vi "thermometer.vi"(1 "upper bound":dbl, 2 "lower bound":dbl) -> (0 "Deg C":dbl)   [LabVIEW 2014]
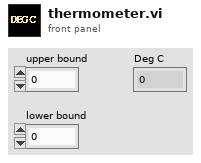
[diagram p1: front panel]
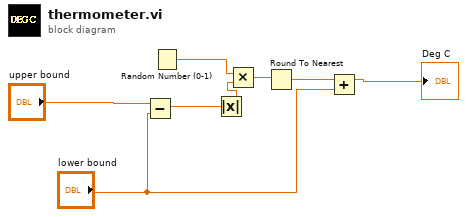
[diagram p0: block diagram]
diagram:
  n1 = Subtract(x="upper bound", y="lower bound") -> (x-y=w5:dbl)
  n2 = Random Number (0-1)() -> (number: 0 to 1=w3:dbl)
  n3 = Absolute Value(x=w5) -> (abs(x)=w4:dbl)
  n4 = Multiply(x=w3, y=w4) -> (x*y=w7:dbl)
  n5 = Round To Nearest(number=w7) -> (nearest integer value=w8:dbl)
  n6 = Add(x=w8, y="lower bound") -> (x+y=→"Deg C":dbl)
